vi "Comm Send and Receive.vi"(4 "Resp Required?":bool, 6 "Timeout (ms)":u32=2000, 8 "error in (no error)":errorcluster, 9 "Data":string, 10 "Name":string, 11 "connection info":T1) -> (0 "error out":errorcluster, 1 "Data":string, 2 "Timed Out?":bool, 3 "connection info":T1)   [LabVIEW 2018, in "NI VeriStand Addon Network Comm Shared.lvlib"]
uses:
  NI VeriStand Addon Network Comm Shared.lvlib
  <vilib>/NI/STM/TCP/TCP Connection Info.ctl
  <vilib>/NI/STM/SubVIs/MetaDataElement.ctl
  _Types/Comm Message.ctl
  <vilib>/NI/STM/TCP/TCP Write Options.ctl
  <vilib>/NI/STM/TCP/TCP Read Options.ctl
  <vilib>/NI/STM/TCP/Write Message (TCP).vi
  Comm Constants.vi
  <vilib>/NI/STM/TCP/Read Message (TCP).vi
  <vilib>/NI/STM/NI STM.lvlib
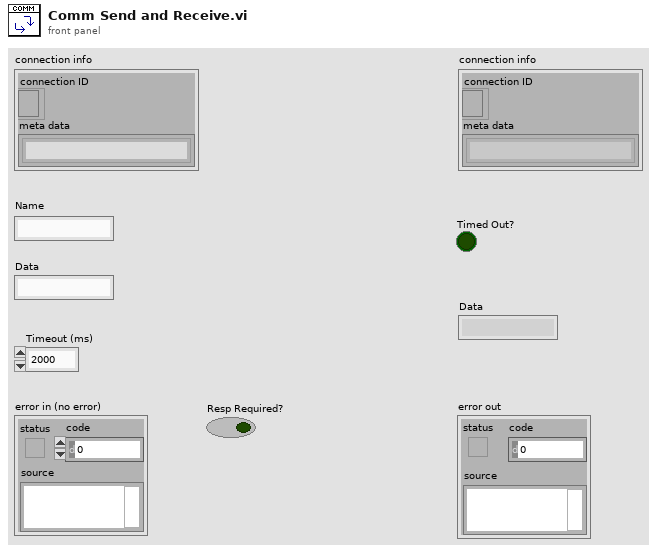
[diagram p1: front panel]
types:
  T1 = typedef "NI STM.lvlib/TCP Connection Info.ctl" = cluster{"connection ID":refnum<k5>, "meta data":T2[]}
  T2 = typedef "NI STM.lvlib/MetaDataElement.ctl" = string
  T3 = typedef "NI STM.lvlib/TCP Write Options.ctl" = cluster{"ignore timeout error":bool, "timeout ms (1000)":i32}
  T4 = typedef "NI VeriStand Addon Network Comm Shared.lvlib/Comm Message.ctl" = cluster{"Timeout":u32, "Resp?":bool, "data":string}
  T5 = typedef "NI STM.lvlib/TCP Read Options.ctl" = cluster{"ignore timeout error":bool, "timeout ms (1000)":i32}
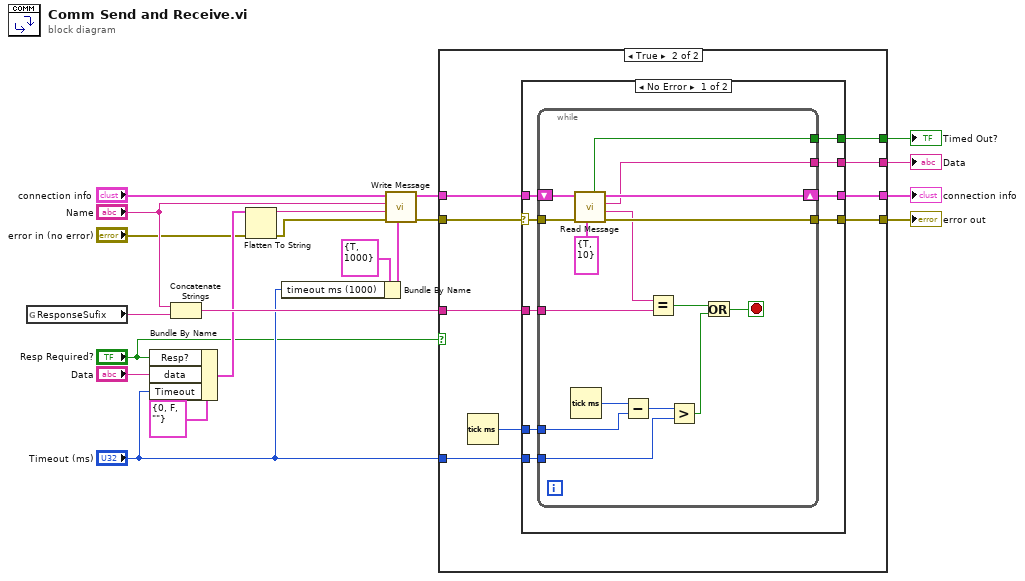
[diagram p0: block diagram]
diagram:
  n1 = global read "Comm Constants.vi" "ResponseSufix"() -> (w11:string)
  n2 = Bundle By Name(cluster=T4 {"Timeout"=0, "Resp?"=FALSE, "data"=""} ("Cluster"), "Resp?"="Resp Required?", "data"="Data", "Timeout"="Timeout (ms)") -> (w9:T4)
  n3 = Concatenate Strings("Name", w11) -> (w16:string)
  n4 = Flatten To String(anything=w9, error in (no error)="error in (no error)") -> (data string=w6:string, error out=w7:errorcluster)  [unwired: 2 in, 1 out]
  n5 = Bundle By Name(cluster=T3 {"ignore timeout error"=TRUE, "timeout ms (1000)"=1000} ("options"), "timeout ms (1000)"="Timeout (ms)") -> (w4:T3)
  n6 = call-poly <vilib>:"Write Message.vi"("options"=w4, "error in"=w7, "data"=w6, "name"="Name", "connection info in"="connection info") -> ("error out"=w12:errorcluster, "connection info out"=w20:T1)  [unwired: 5 in]
  n7 = case shown="True" "Resp Required?" {
    tunnel: w20 -> [w21 w31]
    tunnel: [w22 w30] -> w18
    tunnel: w16 -> [_ w29]
    tunnel: [w21 w27] -> w15
    tunnel: [_ w26] -> w14
    tunnel: [_ w25] -> w13
    tunnel: w12 -> [w22 w24]
    tunnel: "Timeout (ms)" -> [_ w23]
    frame False {
    }
    frame True {
      n8 = Tick Count (ms)() -> (millisecond timer value=w28:u32)
      n9 = case shown="No Error" w24 {
        selector: w24 -> [w32 w58]
        tunnel: w31 -> [w40 w57]
        tunnel: [w39 w58] -> w30
        tunnel: w29 -> [w38 _]
        tunnel: w28 -> [w37 _]
        tunnel: w23 -> [w36 _]
        tunnel: [w35 w57] -> w27
        tunnel: [w34 _] -> w26
        tunnel: [w33 _] -> w25
        frame No Error {
          n10 = while {
            tunnel: w32 -> [w55]
            tunnel: [w54] -> w39
            tunnel: w38 -> [w53]
            tunnel: w37 -> [w51]
            tunnel: w36 -> [w49]
            shift-right: [w45] -> w35
            shift-left: w40 -> [w56]
            tunnel: [w43] -> w34
            tunnel: [w42] -> w33
            stop <- w46 stop-if-true
            n11 = Tick Count (ms)() -> (millisecond timer value=w52:u32)
            n12 = call-poly <vilib>:"Read Message.vi"("options"=T5 {"ignore timeout error"=TRUE, "timeout ms (1000)"=10}, "error in"=w55, "connection info in"=w56) -> ("error out"=w54:errorcluster, "name"=w44:T2, "data string"=w43:string, "connection info out"=w45:T1, "timed out?"=w42:bool)  [unwired: 3 in, 1 out]
            n13 = Subtract(x=w52, y=w51) -> (x-y=w50:u32)
            n14 = Equal?(x=w44, y=w53) -> (x = y?=w47:bool)
            n15 = Greater?(x=w50, y=w49) -> (0:w48:bool)
            n16 = Or(x=w47, y=w48) -> (x .or. y?=w46:bool)
          }
        }
        frame Error {
        }
      }
    }
  }
  "error out" <- w18
  "connection info" <- w15
  "Data" <- w14
  "Timed Out?" <- w13
